vi "Draw CI Band from CI Plots.vi"(8 "error in (no error)":errorcluster, 10 "CI Plots?":bool, 11 "XYGraph in":T1) -> (0 "error out":errorcluster, 3 "XYGraph out":T1)   [LabVIEW 2021, in "AlliGator Decay Fit.lvlib"]
doc: "Connects the last two plots of a XY Graph to draw a CI band around the fitted plot.\n\nThis needs to be used right after the two CI plots have be drawn."
uses:
  AlliGator/Decay Analysis/Decay Fit/AlliGator Decay Fit.lvlib
  Graphs/XY Graph/XY Graph Refnum.ctl
  Graphs/XY Graph/XY Graph Add-Ons.lvlib
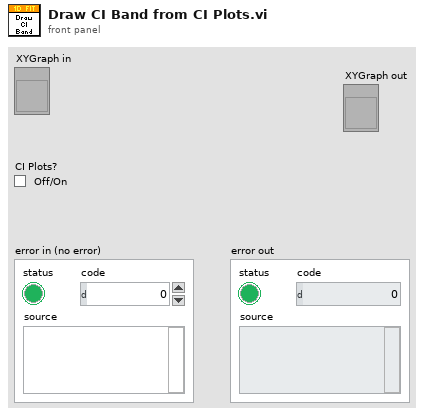
[diagram p1: front panel]
types:
  T1 = typedef "XY Graph Add-Ons.lvlib/XY Graph Refnum.ctl" = refnum<vi>
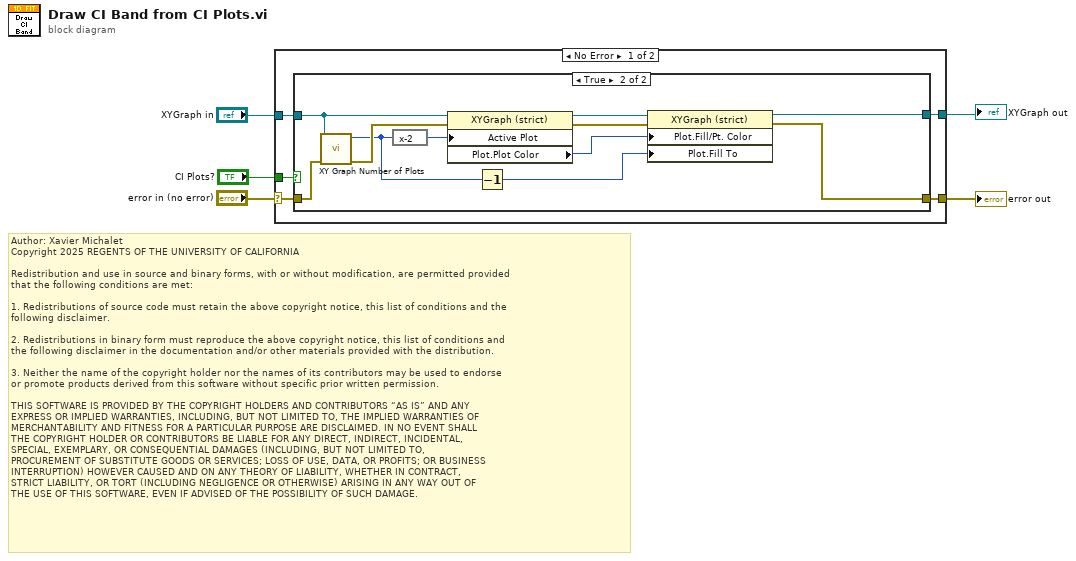
[diagram p0: block diagram]
diagram:
  # "Author: Xavier Michalet\nCopyright 2025 REGENTS OF THE UNIVERSITY OF CALIFORNIA\n\nRedistribution and use in source and binary forms, with or without modification, are permitted provided\nthat the following conditions are met:\n\n1. Redistributions of source code must retain the above copyright notice, this list of conditions and the\nfollowing disclaimer.\n\n2. Redistributions in binary form must reproduce the above copyright notice, this list of conditions and\nthe following disclaimer in the documentation and/or other materials provided with the distribution.\n\n3. Neither the name of the copyright holder nor the names of its contributors may be used to endorse \nor promote products derived from this software without specific prior written permission.\n\nTHIS SOFTWARE IS PROVIDED BY THE COPYRIGHT HOLDERS AND CONTRIBUTORS “AS IS” AND ANY \nEXPRESS OR IMPLIED WARRANTIES, INCLUDING, BUT NOT LIMITED TO, THE IMPLIED WARRANTIES OF\nMERCHANTABILITY AND FITNESS FOR A PARTICULAR PURPOSE ARE DISCLAIMED. IN NO EVENT SHALL\nTHE COPYRIGHT HOLDER OR CONTRIBUTORS BE LIABLE FOR ANY DIRECT, INDIRECT, INCIDENTAL, \nSPECIAL, EXEMPLARY, OR CONSEQUENTIAL DAMAGES (INCLUDING, BUT NOT LIMITED TO, \nPROCUREMENT OF SUBSTITUTE GOODS OR SERVICES; LOSS OF USE, DATA, OR PROFITS; OR BUSINESS\nINTERRUPTION) HOWEVER CAUSED AND ON ANY THEORY OF LIABILITY, WHETHER IN CONTRACT, \nSTRICT LIABILITY, OR TORT (INCLUDING NEGLIGENCE OR OTHERWISE) ARISING IN ANY WAY OUT OF\nTHE USE OF THIS SOFTWARE, EVEN IF ADVISED OF THE POSSIBILITY OF SUCH DAMAGE."
  n1 = case shown="No Error" "error in (no error)" {
    selector: "error in (no error)" -> [w10 w25]
    tunnel: [w8 w25] -> w4
    tunnel: "CI Plots?" -> [w9 _]
    tunnel: "XYGraph in" -> [w7 w24]
    tunnel: [w6 w24] -> w1
    frame No Error {
      n2 = case shown="True" w9 {
        tunnel: w10 -> [w12 w14]
        tunnel: [w12 w15] -> w8
        tunnel: w7 -> [w11 w23]
        tunnel: [w11 w13] -> w6
        frame False {
        }
        frame True {
          n3 = call "XY Graph Number of Plots.vi"("Error In"=w14, "XYGraph in"=w23) -> ("Error Out"=w22:errorcluster, "# Plots"=w17:i32)  [unwired: 8 in]
          n4 = expression code="x-2"(w17) -> (w19:i32)
          n5 = property class="XYGraph (strict)"(reference=w23, error in=w22, "Active Plot"=w19) -> (reference out=w21:T1, error out=w20:errorcluster, "Plot.Plot Color"=w18:u32)
          n6 = Decrement(x=w17) -> (x-1=w16:i32)
          n7 = property class="XYGraph (strict)"(reference=w21, error in=w20, "Plot.Fill/Pt. Color"=w18, "Plot.Fill To"=w16) -> (reference out=w13:T1, error out=w15:errorcluster)
        }
      }
    }
    frame Error {
    }
  }
  "error out" <- w4
  "XYGraph out" <- w1
